vi "Skip Object.vi"(8 "error in (no error)":errorcluster, 10 "Header":T1, 11 "BLF File In":refnum<class "Read Write BLF.lvclass">) -> (0 "error out":errorcluster, 3 "BLF File Out":refnum<class "Read Write BLF.lvclass">)   [LabVIEW 2015, in "Read Write BLF.lvclass"]
doc: "This VI will skip the next object to be read, preparing to advance the file read position.\n\n-------------\nBrian Hoover (Hooovahh)"
uses:
  Read Write BLF.lvclass
  Controls/Cluster - mHeaderBase.ctl
  Controls/Enum - Read Object Types.ctl
  Read Write BLF.lvclass/Read Write BLF.ctl
  <vilib>/Utility/error.llb/Error Cluster From Error Code.vi
  <vilib>/Utility/libraryn.llb/Check if File or Folder Exists.vi
  <vilib>/Utility/file.llb/Application Directory.vi
  <vilib>/ErrorRing/Error Ring.xnode
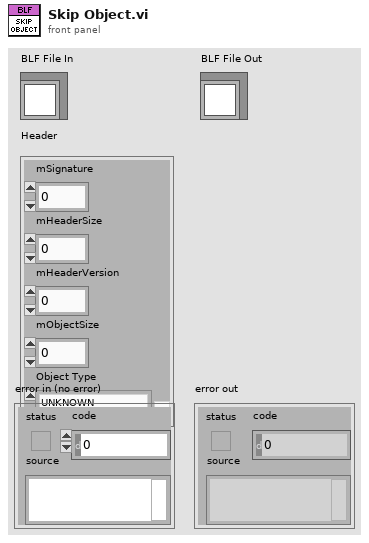
[diagram p1: front panel]
types:
  T1 = typedef "Read Write BLF.lvclass/Cluster - mHeaderBase.ctl" = cluster{"mSignature":u32, "mHeaderSize":u16, "mHeaderVersion":u16, "mObjectSize":u32, "Object Type":T2}
  T2 = typedef "Read Write BLF.lvclass/Enum - Read Object Types.ctl" = enum32{"UNKNOWN", "CAN_MESSAGE", "CAN_ERROR", "CAN_OVERLOAD", "CAN_STATISTIC", "APP_TRIGGER", "ENV_INTEGER", "ENV_DOUBLE", "ENV_STRING", "ENV_DATA", "LOG_CONTAINER", "LIN_MESSAGE", "LIN_CRC_ERROR", "LIN_DLC_INFO", "LIN_RCV_ERROR", "LIN_SND_ERROR", "LIN_SLV_TIMEOUT", "LIN_SCHED_MODCH", "LIN_SYN_ERROR", "LIN_BAUDRATE", "LIN_SLEEP", "LIN_WAKEUP", "MOST_SPY", "MOST_CTRL", "MOST_LIGHTLOCK", "MOST_STATISTIC", "reserved_1", "reserved_2", "reserved_3", "FLEXRAY_DATA", "FLEXRAY_SYNC", "CAN_DRIVER_ERROR", "MOST_PKT", "MOST_PKT2", "MOST_HWMODE", "MOST_REG", "MOST_GENREG", "MOST_NETSTATE", "MOST_DATALOST", "MOST_TRIGGER", "FLEXRAY_CYCLE", "FLEXRAY_MESSAGE", "LIN_CHECKSUM_INFO", "LIN_SPIKE_EVENT", "CAN_DRIVER_SYNC", "FLEXRAY_STATUS", "GPS_EVENT", "FR_ERROR", "FR_STATUS", "FR_STARTCYCLE", "FR_RCVMESSAGE", "REALTIMECLOCK", "AVAILABLE2", "AVAILABLE3", "LIN_STATISTIC", "J1708_MESSAGE", "J1708_VIRTUAL_MSG", "LIN_MESSAGE2", "LIN_SND_ERROR2", "LIN_SYN_ERROR2", "LIN_CRC_ERROR2", "LIN_RCV_ERROR2", "LIN_WAKEUP2", "LIN_SPIKE_EVENT2", "LIN_LONG_DOM_SIG", "APP_TEXT", "FR_RCVMESSAGE_EX", "MOST_STATISTICEX", "MOST_TXLIGHT", "MOST_ALLOCTAB", "MOST_STRESS", "ETHERNET_FRAME", "SYS_VARIABLE", "CAN_ERROR_EXT", "CAN_DRIVER_ERROR_EXT", "LIN_LONG_DOM_SIG2", "MOST_150_MESSAGE", "MOST_150_PKT", "MOST_ETHERNET_PKT", "MOST_150_MESSAGE_FRAGMENT", "MOST_150_PKT_FRAGMENT", "MOST_ETHERNET_PKT_FRAGMENT", "MOST_SYSTEM_EVENT", "MOST_150_ALLOCTAB", "MOST_50_MESSAGE", "MOST_50_PKT", "CAN_MESSAGE2", "LIN_UNEXPECTED_WAKEUP", "LIN_SHORT_OR_SLOW_RESPONSE", "LIN_DISTURBANCE_EVENT", "SERIAL_EVENT", "OVERRUN_ERROR", "EVENT_COMMENT", "WLAN_FRAME", "WLAN_STATISTIC", "MOST_ECL", "GLOBAL_MARKER", "AFDX_FRAME", "AFDX_STATISTIC", "KLINE_STATUSEVENT", "CAN_FD_MESSAGE", "CAN_FD_MESSAGE_64", "ETHERNET_RX_ERROR", "ETHERNET_STATUS", "CAN_FD_ERROR_64", "LIN_SHORT_OR_SLOW_RESPONSE2", "AFDX_STATUS", "AFDX_BUS_STATISTIC"}
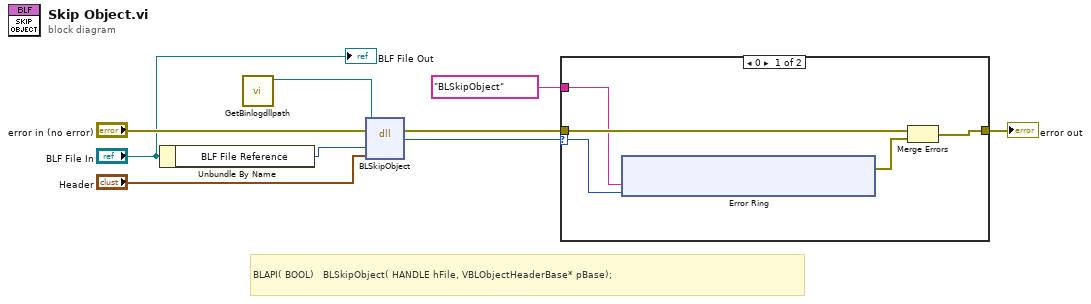
[diagram p0: block diagram]
diagram:
  # "BLAPI( BOOL)   BLSkipObject( HANDLE hFile, VBLObjectHeaderBase* pBase);"
  n1 = Unbundle By Name("BLF File In") -> ("BLF File Reference"=w2:u32)
  n2 = call "GetBinlogdllpath.vi"() -> ("dup path"=w1:path)  [unwired: 11 in]
  n3 = dll-call lib="PTH2Vabs E自开发软件X-CAN项目 X-CAN离线分析平台 V2.2.8.0BLFbinlog.*" fn="BLSkipObject"(path in=w1, error in="error in (no error)", "hFile"=w2, "pBase"="Header") -> (error out=w5:errorcluster, "return type"=w6:i32)  [unwired: 3 in, 1 out]
  n4 = case shown="0" w6 {
    selector: w6 -> [w12 _]
    tunnel: w5 -> [w14 w23]
    tunnel: [w13 w23] -> w4
    tunnel: "BLSkipObject" -> [w11 _]
    frame 0 {
      n5 = xnode "Error Ring"("参数 0"=w11, "参数 1"=w12) -> ("错误输出"=w10:errorcluster)
      n6 = Merge Errors(w14, w10) -> (w13:errorcluster)
    }
    frame Default {
    }
  }
  "error out" <- w4
  "BLF File Out" <- "BLF File In"
